vi "Datasheet Populate Fields West.vi"(6 "System or ALL Combined Fields":T1[](array[typedef]), 7 "Source Parameters":T4, 8 "error in (no error)":errorcluster, 9 "Custom Fields":T1[][](array[typedef]), 10 "Parameters":T4) -> (0 "error out":errorcluster, 2 "Parameters 2":T4)   [LabVIEW 2011]
uses:
  database/Fields/Field Record.ctl
  database/Fields/Field DataTypes.ctl
  database/Fields/Field NextItem.ctl
  Addons/internet/utils/keyedarr.llb/Keyed Array.ctl
  Addons/internet/utils/strutil.llb/Case Matching.ctl
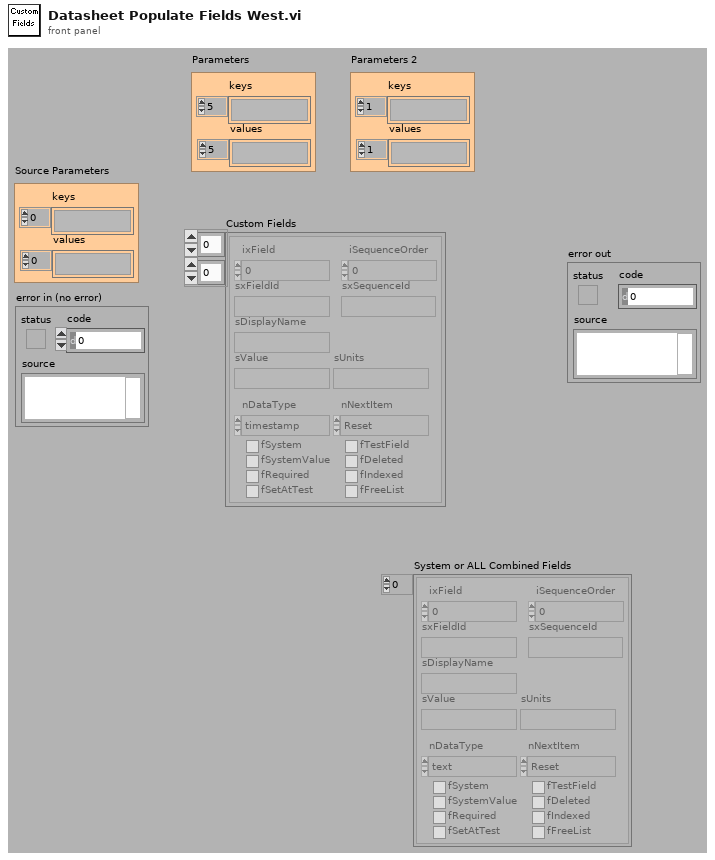
[diagram p1: front panel]
types:
  T1 = typedef "Field Record.ctl" = cluster{"ixField":i32, "iSequenceOrder":i32, "sxFieldId":string, "sxSequenceId":string, "sDisplayName":string, "sValue":string, "sUnits":string, "nDataType":T2, "nNextItem":T3, "fSystem":bool, "fSystemValue":bool, "fRequired":bool, "fSetAtTest":bool, "fTestField":bool, "fDeleted":bool, "fIndexed":bool, "fFreeList":bool}
  T2 = typedef "Field DataTypes.ctl" = enum32{"text", "numeric", "list", "timestamp", "boolean"}
  T3 = typedef "Field NextItem.ctl" = enum32{"Reset", "Retain", "Auto-Increment"}
  T4 = typedef "Keyed Array.ctl" = cluster{"keys":string[], "values":string[]}
  T5 = typedef "Case Matching.ctl" = enum16{"a != A", "a == A", "system"}
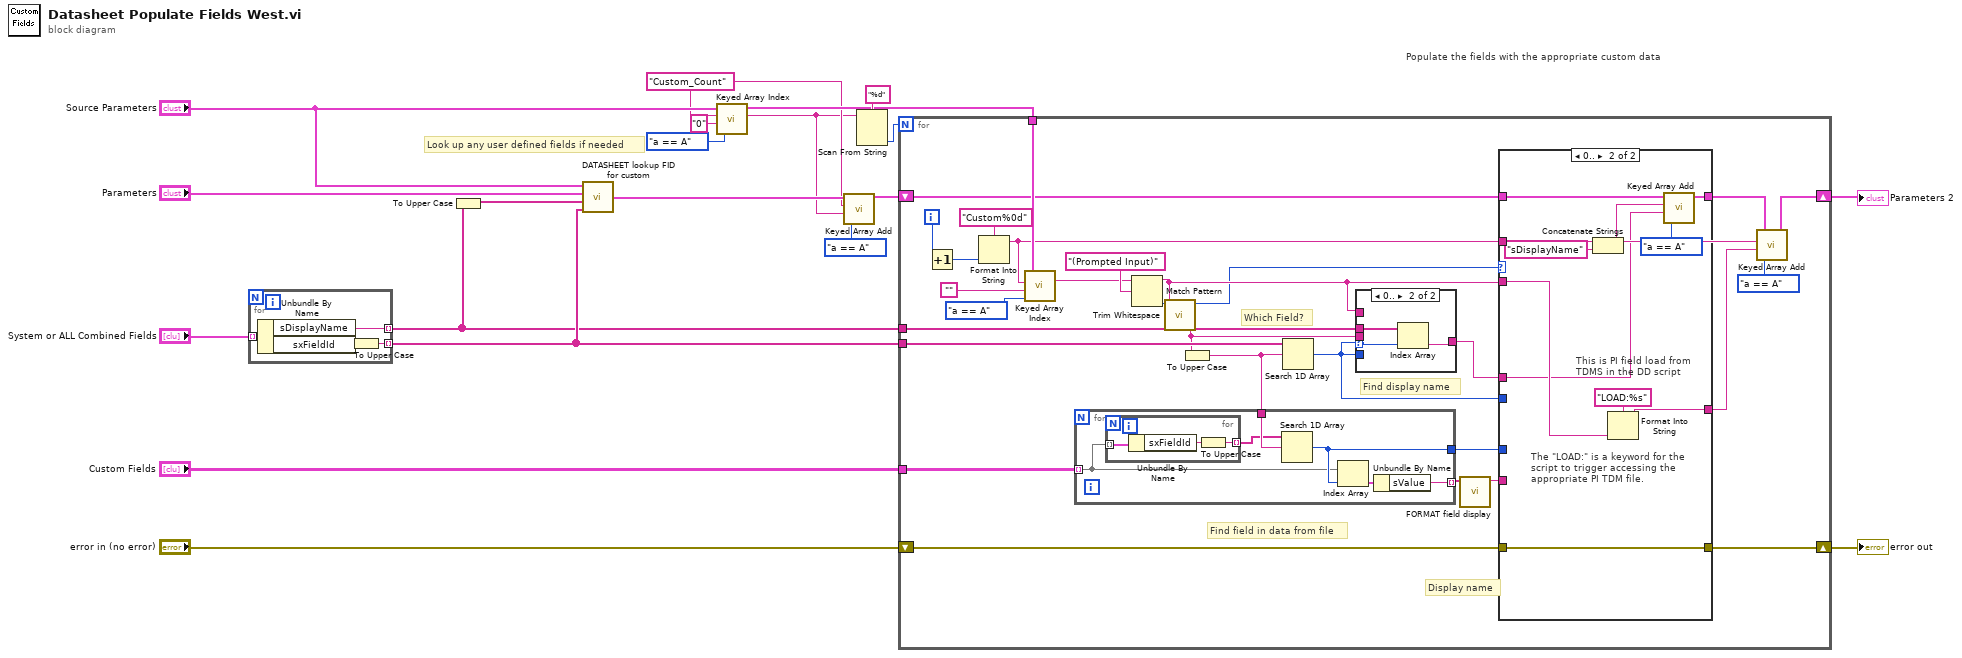
[diagram p0: block diagram]
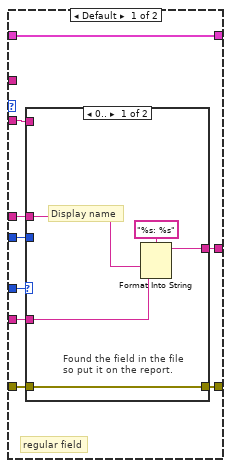
[diagram p3: hidden frame]
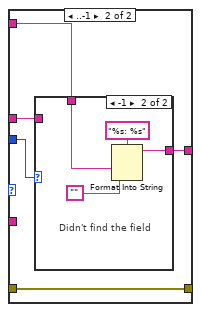
[diagram p4: hidden frame]
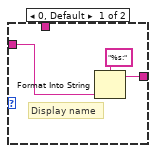
[diagram p5: hidden frame]
diagram:
  w4 = "Custom_Count" ("format string")
  # "Look up any user defined fields if needed"
  # "Populate the fields with the appropriate custom data"
  n1 = for {
    tunnel: "System or ALL Combined Fields" -> [w24] mode=indexing
    tunnel: [w21] -> w11 mode=indexing
    tunnel: [w22] -> w10 mode=indexing
    n2 = Unbundle By Name(w24) -> ("sDisplayName"=w22:string, "sxFieldId"=w23:string)
    n3 = To Upper Case(1:w23) -> (0:w21:string)
  }
  n4 = To Upper Case(1:w10) -> (0:w9:string[])
  n5 = call "DATASHEET lookup FID for custom.vi"("sxFieldId"=w11, "Display Names"=w9, "Modified Report Parameters"="Parameters", "Original Parameters"="Source Parameters") -> ("Report Parameters"=w6:T4)
  n6 = call "Keyed Array Index.vi"("case matching (sensitive)"=Case_Matching."a == A", "default value"="0", "key"=w4, "array in"="Source Parameters") -> ("value"=w3:string, "duplicate array"=w13:T4)  [unwired: 2 out]
  n7 = call "Keyed Array Add.vi"("case matching (sensitive)"=Case_Matching."a == A", "value"=w3, "key"=w4, "array in"=w6) -> ("array out"=w5:T4)  [unwired: 3 out]
  n8 = Scan From String(format string="%d", input string=w3) -> (output 1=w14:i32)  [unwired: 2 in, 4 out]
  n9 = for {
    N: w14 -> [_]
    shift-right: [w46] -> w19
    shift-left: w5 -> [w27]
    tunnel: w11 -> [w38]
    tunnel: "Custom Fields" -> [w52]
    shift-right: [w50] -> w20
    shift-left: "error in (no error)" -> [w51]
    tunnel: w10 -> [w42]
    tunnel: w13 -> [w36]
    i -> [w47]
    # "Display name"
    # "Which Field?"
    # "Find field in data from file"
    # "Find display name"
    n10 = Increment(x=w47) -> (x+1=w39:i32)
    n11 = Format Into String(format string="Custom%0d", w39) -> (resulting string=w25:string)  [unwired: 2 in, 1 out]
    n12 = call "Keyed Array Index.vi"("case matching (sensitive)"=Case_Matching."a == A", "default value"="", "key"=w25, "array in"=w36) -> ("value"=w34:string)  [unwired: 3 out]
    n13 = Match Pattern(string=w34, regular expression="(Prompted Input)") -> (before substring=w33:string, offset past match=w32:i32)  [unwired: 3 out]
    n14 = call <vilib>:"Trim Whitespace.vi"("string"=w33) -> ("trimmed string"=w28:string)  [unwired: 1 in]
    n15 = To Upper Case(1:w28) -> (0:w37:string)
    n16 = for {
      tunnel: w52 -> [w56] mode=indexing
      tunnel: [w58] -> w41
      tunnel: w37 -> [w57]
      tunnel: [w53] -> w30 mode=indexing
      n17 = for {
        tunnel: w56 -> [w61] mode=indexing
        tunnel: [w59] -> w55 mode=indexing
        n18 = Unbundle By Name(w61) -> ("sxFieldId"=w60:string)
        n19 = To Upper Case(1:w60) -> (0:w59:string)
      }
      n20 = Search 1D Array(1D array=w55, element=w57) -> (index of element=w58:i32)  [unwired: 1 out]
      n21 = Index Array(array=w56, index=w58) -> (element=w54:T1)
      n22 = Unbundle By Name(w54) -> ("sValue"=w53:string)
    }
    n23 = Search 1D Array(1D array=w38, element=w37) -> (index of element=w31:i32)  [unwired: 1 out]
    n24 = case shown="0.." w31 {
      selector: w31 -> [_ w64]
      tunnel: w42 -> [_ w65]
      tunnel: [w62 w63] -> w40
      tunnel: w31 -> [_ _]
      tunnel: w33 -> [w62 _]
      tunnel: w28 -> [_ _]
      frame Default {
      }
      frame 0.. {
        n25 = Index Array(array=w65, index=w64) -> (element=w63:string)
      }
    }
    n26 = call "FORMAT field display.vi"("strings"=w30) -> ("String"=w29:string)  [unwired: 10 out]
    n27 = case shown="0.." w32 {
      tunnel: [w74 w101] -> w45
      tunnel: w51 -> [w73 w100]
      tunnel: [w72 w100] -> w50
      tunnel: w40 -> [w71 w92]
      tunnel: w41 -> [w67 _]
      tunnel: w33 -> [w70 w99]
      tunnel: w31 -> [w69 _]
      tunnel: w29 -> [w68 _]
      tunnel: w27 -> [w66 w98]
      tunnel: [w66 w97] -> w26
      tunnel: w25 -> [_ w95]
      frame Default {
        # "regular field"
        n28 = case shown="0.." w67 {
          tunnel: [w78 w84] -> w74
          tunnel: w71 -> [w76 w80]
          tunnel: w73 -> [w77 w83]
          tunnel: [w77 w83] -> w72
          tunnel: w70 -> [_ w82]
          tunnel: w69 -> [_ w81]
          tunnel: w68 -> [w75 _]
          frame 0.. {
            # "Display name"
            # "Found the field in the file\nso put it on the report."
            n29 = Format Into String(format string="%s: %s", w76, w75) -> (resulting string=w78:string)  [unwired: 2 in, 1 out]
          }
          frame ..-1 {
            n30 = case shown="-1" w81 {
              tunnel: [w86 w90] -> w84
              tunnel: w82 -> [_ w89]
              tunnel: w80 -> [w87 _]
              frame 0, Default {
                # "Display name"
                n31 = Format Into String(format string="%s:", w87) -> (resulting string=w86:string)  [unwired: 2 in, 1 out]
              }
              frame -1 {
                # "Didn't find the field"
                n32 = Format Into String(format string="%s: %s", w89, "") -> (resulting string=w90:string)  [unwired: 2 in, 1 out]
              }
            }
          }
        }
      }
      frame 0.. {
        # "This is PI field load from\nTDMS in the DD script"
        # "The \"LOAD:\" is a keyword for the\nscript to trigger accessing the\nappropriate PI TDM file."
        n33 = Concatenate Strings(w95, "sDisplayName" ("string")) -> (w93:string)
        n34 = Format Into String(format string="LOAD:%s", w99) -> (resulting string=w101:string)  [unwired: 2 in, 1 out]
        n35 = call "Keyed Array Add.vi"("case matching (sensitive)"=Case_Matching."a == A", "value"=w92, "key"=w93, "array in"=w98) -> ("array out"=w97:T4)  [unwired: 3 out]
      }
    }
    n36 = call "Keyed Array Add.vi"("case matching (sensitive)"=Case_Matching."a == A", "value"=w45, "key"=w25, "array in"=w26) -> ("array out"=w46:T4)  [unwired: 3 out]
  }
  "error out" <- w20
  "Parameters 2" <- w19
